vi "CalibrationInfo.vi"(0 "refnum":refnum<file>, 11 "offset":i32) -> (4 "dup refnum":refnum<file>, 10 "blank":string)   [LabVIEW 2022 SP3]
panel:
  out "Atten (dB)":sgl
  out "Votage scaling":T1
  out "Gain (dB)":sgl
  out "Digitizer (dB)":sgl
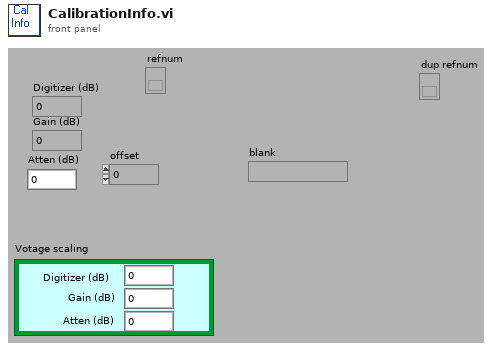
[diagram p1: front panel]
types:
  T1 = cluster{"Digitizer (dB)":sgl, "Gain (dB)":sgl, "Atten (dB)":sgl}
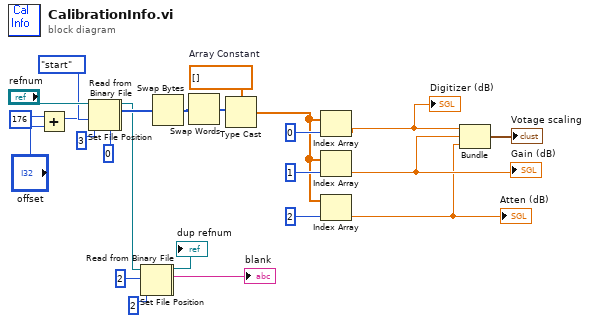
[diagram p0: block diagram]
diagram:
  w9 = sgl[] []  # Array Constant
  n1 = Add(x=176 ("pos offset (0)"), y="offset") -> (x+y=w18:i32)
  n2 = Set File Position(offset (in bytes) (0)=w18, refnum="refnum", from (0:start)=enum16{"start", "end", "current"}."start" ("pos mode (0:2)")) -> (refnum out=w15:refnum<file>, error out=w14:errorcluster)  [unwired: 1 in]
  n3 = Read from Binary File(5:0 ("byte stream type"), 8:w14, 10:3 ("count"), 11:w15) -> (2:w5:i32[], 3:w4:refnum<file>)  [unwired: 4 out]
  n4 = Set File Position(refnum=w4, from (0:start)=2) -> (refnum out=w17:refnum<file>, error out=w16:errorcluster)  [unwired: 1 in, 1 out]
  n5 = Read from Binary File(8:w16, 10:2 ("count"), 11:w17) -> (2:→"blank":string, 3:→"dup refnum":refnum<file>)  [unwired: 5 out]
  n6 = Swap Bytes(anything=w5) -> (byte swapped=w10:i32[])
  n7 = Swap Words(1:w10) -> (0:w8:i32[])
  n8 = Type Cast(type=w9, x=w8) -> (*(type *) &x=w2:sgl[])
  n9 = Index Array(array=w2, index=0) -> (element=w7:sgl)
  "Digitizer (dB)" <- w7
  n10 = Index Array(array=w2, index=1) -> (element=w6:sgl)
  "Gain (dB)" <- w6
  n11 = Index Array(array=w2, index=2) -> (element=w1:sgl)
  "Atten (dB)" <- w1
  n12 = Bundle(w7, w6, w1) -> (→"Votage scaling":cluster{sgl, sgl, sgl})  [unwired: 1 out]
